vi "Index_Array_2D_Element.vi"(9 "Index Array 2D":i8[][](array[numeric])=[[0, 4, -3], [1, 5, -4], [2, -1, -5], [3, -2, 100]], 10 "Indexs IA":T1) -> (2 "Value":i8)   [LabVIEW 2018]
uses:
  Controls/Rows_Columns.ctl
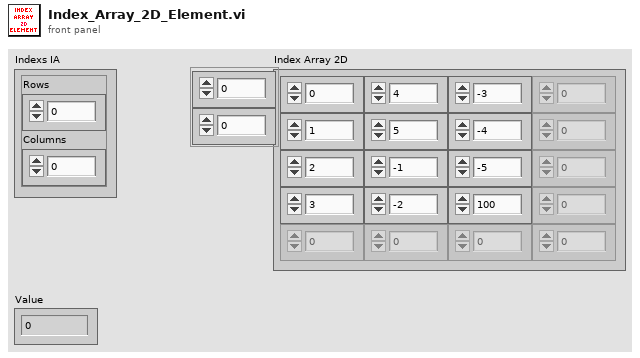
[diagram p1: front panel]
types:
  T1 = typedef "Rows_Columns.ctl" = cluster{"Rows":i32, "Columns":i32}
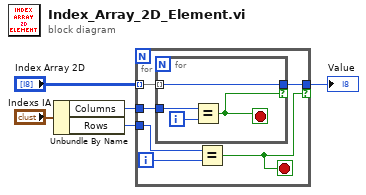
[diagram p0: block diagram]
diagram:
  n1 = Unbundle By Name("Indexs IA") -> ("Columns"=w1:i32, "Rows"=w2:i32)
  n2 = for {
    tunnel: "Index Array 2D" -> [w11] mode=indexing
    tunnel: [w10] -> w4 if=w6
    tunnel: w1 -> [w9]
    tunnel: w2 -> [w8]
    i -> [w7]
    stop <- w6 stop-if-true
    n3 = for {
      tunnel: w11 -> [w15] mode=indexing
      tunnel: [w15] -> w10 if=w12
      tunnel: w9 -> [w13]
      i -> [w14]
      stop <- w12 stop-if-true
      n4 = Equal?(x=w13, y=w14) -> (x = y?=w12:bool)
    }
    n5 = Equal?(x=w8, y=w7) -> (x = y?=w6:bool)
  }
  "Value" <- w4
